vi "Configure Filter.vi"(7 "Enable Filter  (T: Enable)":bool=TRUE, 8 "error in (no error)":errorcluster, 9 "Number of Filter Readings (3)":u32=3, 10 "Filter Type  (0: Repeating)":u16(ring) items=["Repeating", "Moving"], 11 "VISA resource name":refnum<visa-resource-name>) -> (0 "error out":errorcluster, 3 "VISA resource name out":refnum<visa-resource-name>)   [LabVIEW 2020, in "Keithley 24XX.lvlib"]
doc: "Configures the measurement filter, including the number of readings averaged the type of filter applied."
uses:
  <instrlib>/Keithley 24XX/Keithley 24XX.lvlib
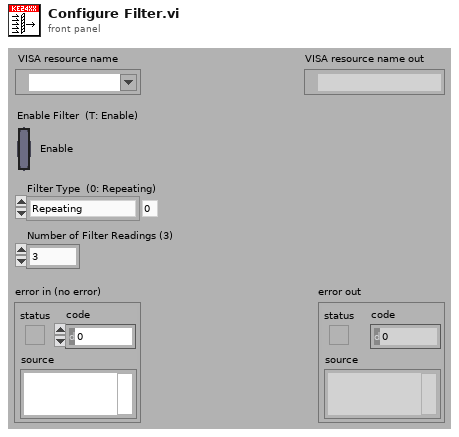
[diagram p1: front panel]
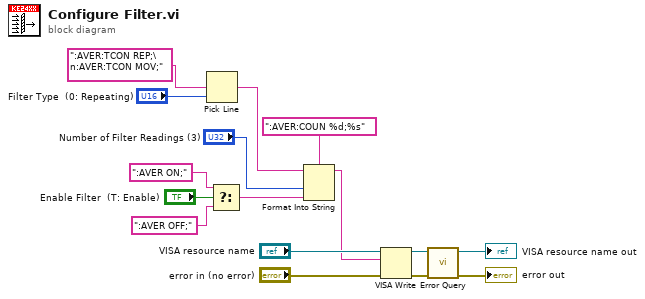
[diagram p0: block diagram]
diagram:
  n1 = Pick Line(multi-line string=":AVER:TCON REP;\n:AVER:TCON MOV;", line index="Filter Type  (0: Repeating)") -> (output string=w3:string)  [unwired: 1 in]
  n2 = Select(t=":AVER ON;", s="Enable Filter  (T: Enable)", f=":AVER OFF;") -> (s? t:f=w5:string)
  n3 = Format Into String(format string=":AVER:COUN %d;%s", initial string=w3, "Number of Filter Readings (3)", w5) -> (resulting string=w1:string)  [unwired: 1 in, 1 out]
  n4 = VISA Write(VISA resource name="VISA resource name", write buffer=w1, error in (no error)="error in (no error)") -> (VISA resource name out=w12:refnum<visa-resource-name>, error out=w11:errorcluster)  [unwired: 1 out]
  n5 = call <instrlib>:"Error Query.vi"("error in (no error)"=w11, "VISA resource name"=w12) -> ("error out"=→"error out":errorcluster, "VISA resource name out"=→"VISA resource name out":refnum<visa-resource-name>)  [unwired: 6 in, 2 out]
